vi "solar_cfg Get Keys.vi"(0 "Config Refnum":refnum<data-value>, 1 "Section":string, 11 "error in (no error)":errorcluster) -> (4 "dup Config Refnum":refnum<data-value>, 6 "Sections":string[](array[string]), 8 "Keys":string[](array[string]), 15 "error out":errorcluster)   [LabVIEW 2018]
doc: "This VI gets all sections and keys from the configuration file reference."
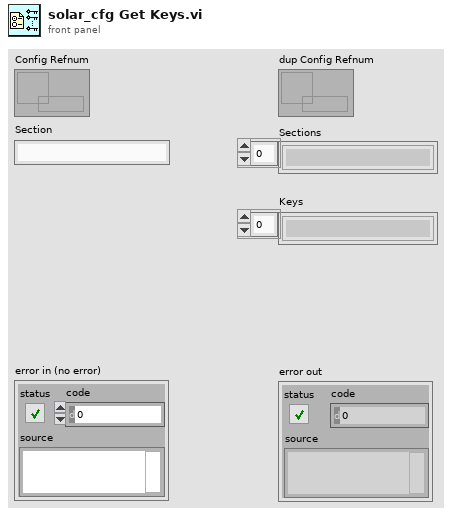
[diagram p1: front panel]
types:
  T1 = cluster{"Dirty":bool, "Semaphore":refnum<queue>, "Sections":cluster{"Section":string, "kvc":string[][]}[], "Path":path}
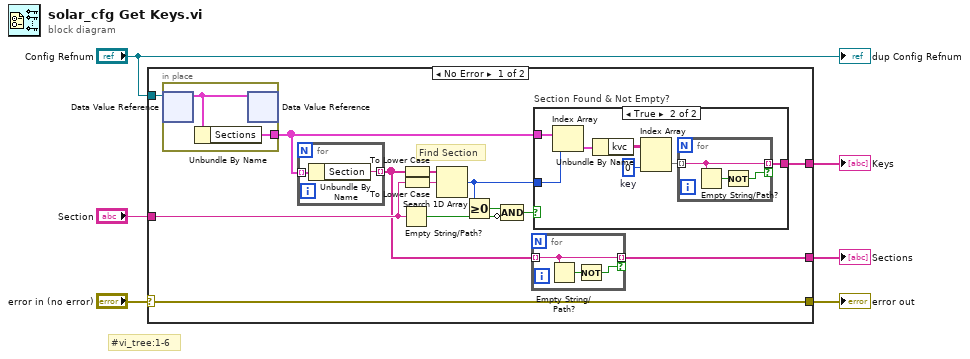
[diagram p0: block diagram]
diagram:
  # "#vi_tree:1-6"
  n1 = case shown="No Error" "error in (no error)" {
    selector: "error in (no error)" -> [w10 w37]
    tunnel: [w10 w37] -> w5
    tunnel: "Section" -> [w19 _]
    tunnel: "Config Refnum" -> [w8 _]
    tunnel: [w7 _] -> w3
    tunnel: [w11 _] -> w2
    frame No Error {
      # "Find Section"
      n2 = in-place {
        in-place-border: [w20] -> w9
        n3 = in-place-dvr #1(w8) -> (w21:T1)  [unwired: 1 out]
        n4 = Unbundle By Name(w21) -> ("Sections"=w20:cluster{"Section":string, "kvc":string[][]}[])
        n5 = in-place-dvr #1(w21) -> ()  [unwired: 2 out]
      }
      n6 = for {
        tunnel: w9 -> [w33] mode=indexing
        tunnel: [w32] -> w12 mode=indexing
        n7 = Unbundle By Name(w33) -> ("Section"=w32:string)
      }
      n8 = Empty String/Path?(string/path=w19) -> (empty?=w14:bool)
      n9 = To Lower Case(string=w12) -> (all lower case string=w17:string[])
      n10 = To Lower Case(string=w19) -> (all lower case string=w18:string)
      n11 = Search 1D Array(1D array=w17, element=w18) -> (index of element=w13:i32)  [unwired: 1 in]
      n12 = Greater Or Equal To 0?(x=w13) -> (x >= 0?=w16:bool)
      n13 = Compound Arithmetic op=AND(w16, invert w14) -> (w15:bool)
      n14 = for {
        tunnel: w12 -> [w36] mode=indexing
        tunnel: [w36] -> w11 mode=indexing if=w34
        n15 = Empty String/Path?(string/path=w36) -> (empty?=w35:bool)
        n16 = Not(x=w35) -> (.not. x?=w34:bool)
      }
      n17 = case "Section Found & Not Empty?" shown="True" w15 {
        tunnel: w9 -> [_ w28]
        tunnel: w13 -> [_ w27]
        tunnel: [_ w25] -> w7
        frame False {
        }
        frame True {
          w23 = 0  # key
          n18 = Index Array(array=w28, index=w27) -> (element=w26:cluster{"Section":string, "kvc":string[][]})
          n19 = Unbundle By Name(w26) -> ("kvc"=w24:string[][])
          n20 = Index Array(array=w24, index (col)=w23) -> (element=w22:string[])  [unwired: 1 in]
          n21 = for {
            tunnel: [w29] -> w25 mode=indexing if=w30
            tunnel: w22 -> [w29] mode=indexing
            n22 = Empty String/Path?(string/path=w29) -> (empty?=w31:bool)
            n23 = Not(x=w31) -> (.not. x?=w30:bool)
          }
        }
      }
    }
    frame Error {
    }
  }
  "error out" <- w5
  "Keys" <- w3
  "Sections" <- w2
  "dup Config Refnum" <- "Config Refnum"
